vi "RootDoesntExist.vi"(11 "base path in":path) -> (3 "String":string)   [LabVIEW 2018]
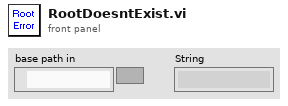
[diagram p1: front panel]
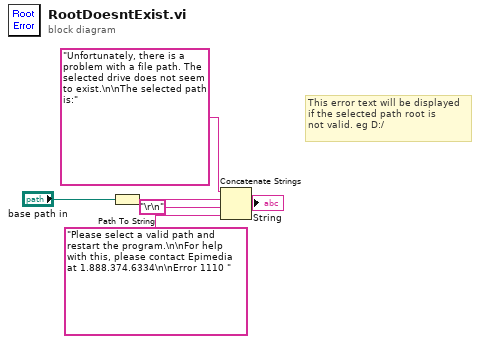
[diagram p0: block diagram]
diagram:
  # "This error text will be displayed\nif the selected path root is \nnot valid. eg D:/"
  n1 = Path To String(path="base path in") -> (string=w3:string)
  n2 = Concatenate Strings("Unfortunately, there is a problem with a file path. The selected drive does not seem to exist.\n\nThe selected path is:", w3, "\r\n", "Please select a valid path and restart the program.\n\nFor help with this, please contact Epimedia at 1.888.374.6334\n\nError 1110 " ("string")) -> (→"String":string)
